vi "Insert Error.vi"(0 "error handler in":refnum<class "TLB` Error Handler.lvclass">, 5 "remaining system actions":string[](array[string]), 11 "captured error in":errorcluster) -> (4 "error handler out":refnum<class "TLB` Error Handler.lvclass">)   [LabVIEW 2026, in "Synchronize AWS S3 Content.lvlib" / "TLB` Error Handler.lvclass"]
uses:
  Error Handler/TLB` Error Handler.lvclass
  Error Handler/TLB` Error Handler.lvclass/TLB` Error Handler.ctl
  <vilib>/regexp/Match Regular Expression.xnode
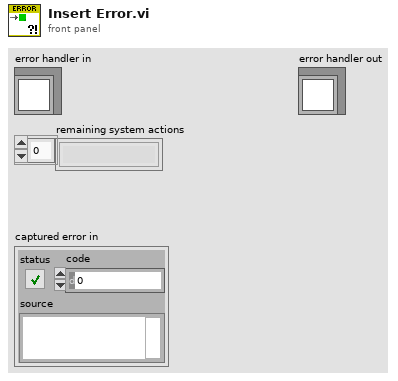
[diagram p1: front panel]
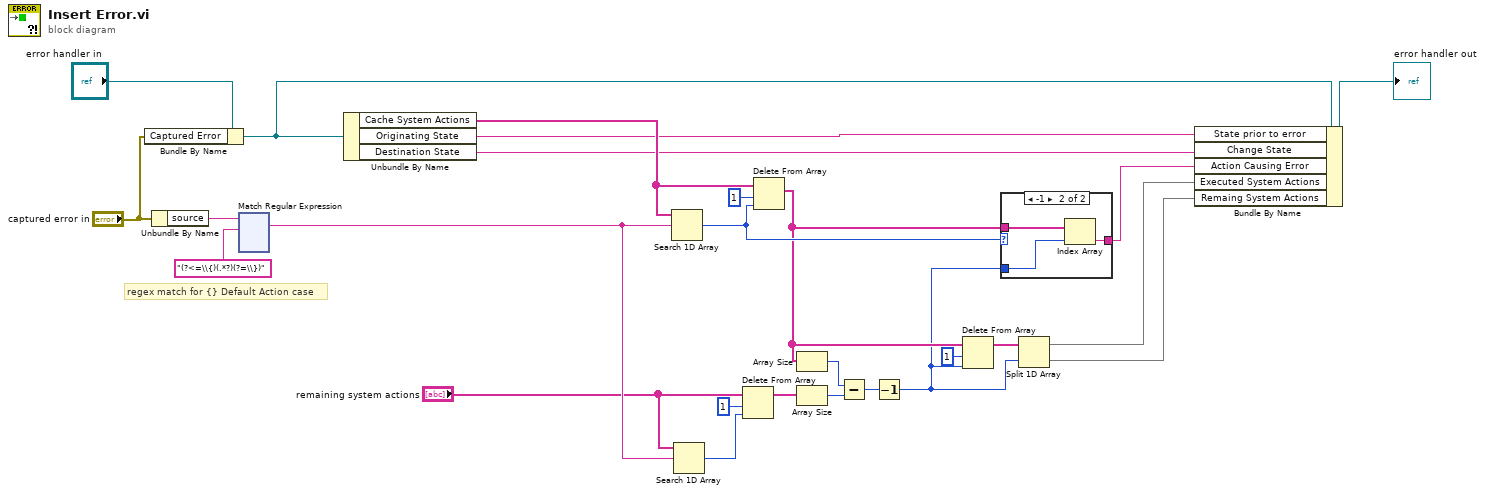
[diagram p0: block diagram]
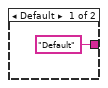
[diagram p2: hidden frame]
diagram:
  # "regex match for {} Default Action case"
  n1 = Bundle By Name(cluster="error handler in", "Captured Error"="captured error in") -> (w12:refnum<class "TLB` Error Handler.lvclass">)
  n2 = Unbundle By Name("captured error in") -> ("source"=w26:string)
  n3 = xnode "Match Regular Expression"("input string"=w26, "regular expression"="(?<=\\{)(.*?)(?=\\})") -> ("whole match"=w18:string)  [unwired: 4 in, 4 out]
  n4 = Unbundle By Name(w12) -> ("Cache System Actions"=w23:string[], "Originating State"=w2:string, "Destination State"=w1:string)
  n5 = Search 1D Array(1D array=w23, element=w18) -> (index of element=w16:i32)  [unwired: 1 in]
  n6 = Search 1D Array(1D array="remaining system actions", element=w18) -> (index of element=w20:i32)  [unwired: 1 in]
  n7 = Delete From Array(array="remaining system actions", length=1, index=w20) -> (array with subset deleted=w17:string[])  [unwired: 1 out]
  n8 = Delete From Array(array=w23, length=1, index=w16) -> (array with subset deleted=w7:string[])  [unwired: 1 out]
  n9 = Array Size(array=w7) -> (size(s)=w22:i32)
  n10 = Array Size(array=w17) -> (size(s)=w21:i32)
  n11 = Subtract(x=w22, y=w21) -> (x-y=w4:i32)
  n12 = Decrement(x=w4) -> (x-1=w3:i32)
  n13 = Delete From Array(array=w7, length=1, index=w3) -> (array with subset deleted=w6:string[])  [unwired: 1 out]
  n14 = case shown="-1" w16 {
    tunnel: w7 -> [_ w30]
    tunnel: ["Default" ("String") w29] -> w11
    tunnel: w3 -> [_ w28]
    frame Default {
    }
    frame -1 {
      n15 = Index Array(array=w30, index=w28) -> (element=w29:string)
    }
  }
  n16 = Split 1D Array(array=w6, index=w3) -> (first subarray=w10:string[], second subarray=w9:string[])
  n17 = Bundle By Name(cluster=w12, "State prior to error"=w2, "Change State"=w1, "Action Causing Error"=w11, "Executed System Actions"=w10, "Remaing System Actions"=w9) -> (→"error handler out":refnum<class "TLB` Error Handler.lvclass">)
